vi "4.4.vi"(1 "数值":dbl) -> (0 "数值 2":i32)   [LabVIEW 2017]
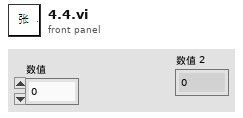
[diagram p1: front panel]
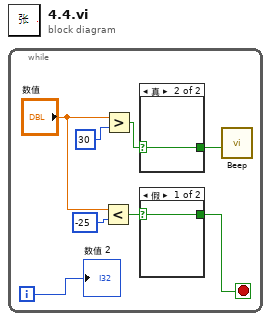
[diagram p0: block diagram]
diagram:
  n1 = while {
    i -> [w1]
    stop <- w7 stop-if-true
    n2 = Less?(x="数值", y=-25) -> (x < y?=w5:bool)
    n3 = Greater?(x="数值", y=30) -> (0:w6:bool)
    n4 = case shown="真" w6 {
      selector: w6 -> [w11 w12]
      tunnel: [w11 w12] -> w8
      frame False {
      }
      frame True {
      }
    }
    n5 = case shown="假" w5 {
      selector: w5 -> [w9 w10]
      tunnel: [w9 w10] -> w7
      frame False {
      }
      frame True {
      }
    }
    n6 = call <vilib>:"Beep.vi"("use system alert? (T)"=w8) -> ()  [unwired: 11 in]
    "数值 2" <- w1
  }
